vi "getAllModels.vi"(3 "len":i32=1024, 5 "错误输入（无错误）":errorcluster) -> (0 "return":i32, 1 "modelNames":string, 2 "错误输出":errorcluster)   [LabVIEW 2013, in "EM_CVx.lvlib"]
uses:
  EM_CVx.lvlib
  library/moverLibrary_x86.dll
  library/moverLibrary_x64.dll
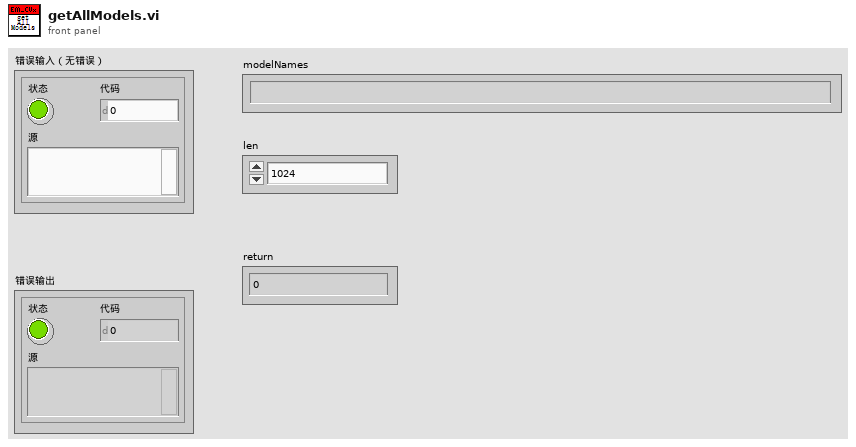
[diagram p1: front panel]
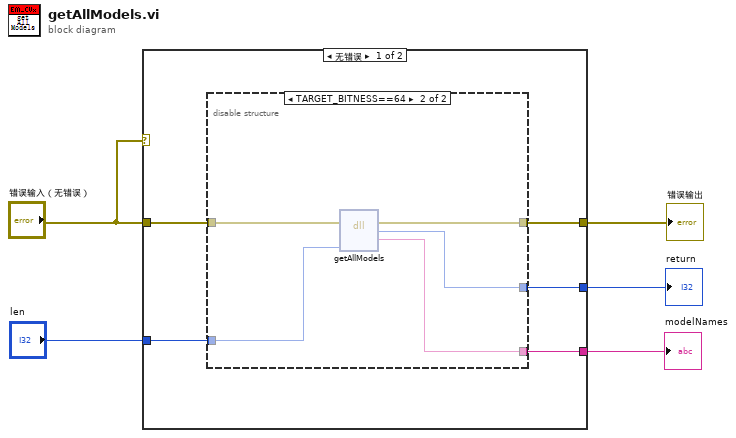
[diagram p0: block diagram]
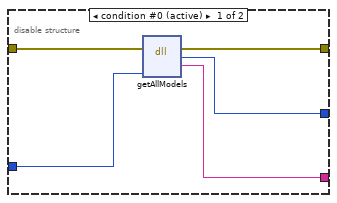
[diagram p2: hidden frame]
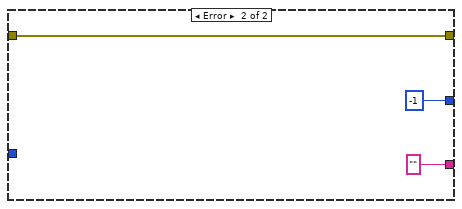
[diagram p3: hidden frame]
diagram:
  n1 = case shown="无错误" "错误输入（无错误）" {
    tunnel: "错误输入（无错误）" -> [w10 w23]
    tunnel: "len" -> [w9 _]
    tunnel: [w8 w23] -> w4
    tunnel: [w7 -1 ("state")] -> w2
    tunnel: [w6 "" ("modelNames")] -> w1
    frame No Error {
      n2 = disable-structure shown="TARGET_BITNESS==64" {
        disable-tunnel: w10 -> [w15 w20]
        disable-tunnel: w9 -> [w14 w18]
        disable-tunnel: [w13 w19] -> w8
        disable-tunnel: [w12 w17] -> w7
        disable-tunnel: [w11 w16] -> w6
        frame condition #0 (active) {
          n3 = dll-call lib="E:/5-mover/4-labView/EM_CVx_2013/library/moverLibrary_x86.dll" fn="getAllModels"(error in=w15, "len"=w14) -> (error out=w13:errorcluster, "return"=w12:i32, "modelNames"=w11:string)  [unwired: 4 in, 1 out]
        }
        frame condition #1 {
          n4 = dll-call lib="E:/5-mover/4-labView/EM_CVx_2013/library/moverLibrary_x64.dll" fn="getAllModels"(error in=w20, "len"=w18) -> (error out=w19:errorcluster, "return"=w17:i32, "modelNames"=w16:string)  [unwired: 4 in, 1 out]
        }
      }
    }
    frame Error {
    }
  }
  "错误输出" <- w4
  "return" <- w2
  "modelNames" <- w1
